vi "setValue.vi"(8 "error in (no error)":errorcluster, 10 "value":variant, 11 "type.ImageData":refnum<class "type.ImageData.lvclass">) -> (0 "error out":errorcluster, 3 "type.ImageData out":refnum<class "type.ImageData.lvclass">)   [LabVIEW 2015, in "type.ImageData.lvclass"]
uses:
  type.ImageData.lvclass
  type.ImageData.lvclass/type.ImageData.ctl
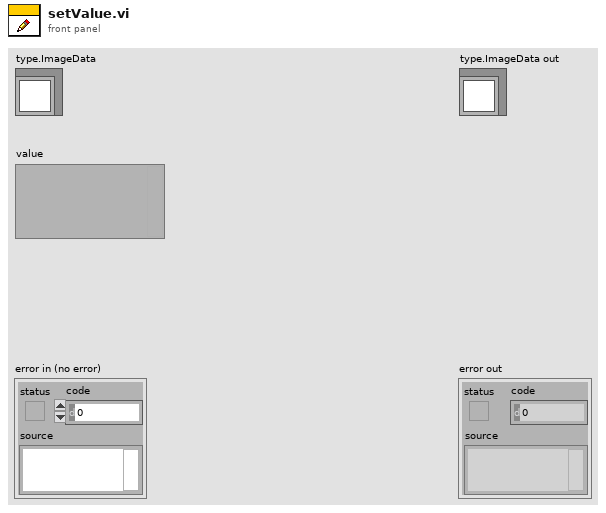
[diagram p1: front panel]
types:
  T1 = typedef "imagedata.ctl" = cluster{"image type":i32, "image depth":i32, "image":u8[], "mask":u8[], "colors":u32[], "Rectangle":cluster{"left":i16, "top":i16, "right":i16, "bottom":i16}}
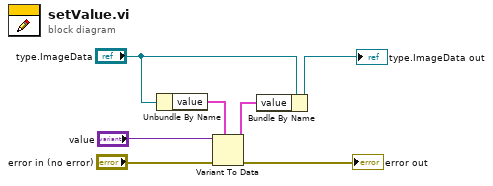
[diagram p0: block diagram]
diagram:
  n1 = Unbundle By Name("type.ImageData") -> ("value"=w4:T1)
  n2 = Variant To Data(error in="error in (no error)", type=w4, Variant="value") -> (data=w3:T1, error out=→"error out":errorcluster)
  n3 = Bundle By Name(cluster="type.ImageData", "value"=w3) -> (→"type.ImageData out":refnum<class "type.ImageData.lvclass">)
